vi "Create StateMachine.vi"(5 "statemachine in":refnum<class "statemachine.lvclass">, 8 "error in (no error)":errorcluster) -> (0 "error out":errorcluster, 3 "statemachine out":refnum<class "statemachine.lvclass">)   [LabVIEW 2020, in "eos.lvlib" / "statemachine.lvclass"]
uses:
  statemachine.lvclass
  interfaces/state/state.lvclass
  interfaces/initialization/initializable.lvclass
  C:/Projects/LVOS/EngineeringOS/source/interfaces/state/state.lvclass
  interfaces/data/data.lvclass
  statemachine.lvclass/statemachine.ctl
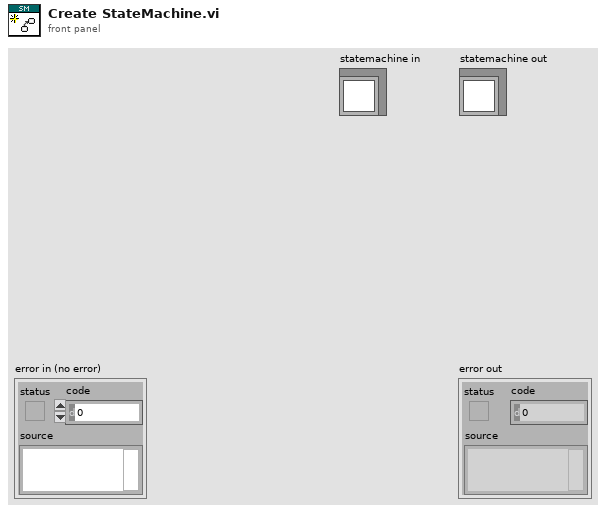
[diagram p1: front panel]
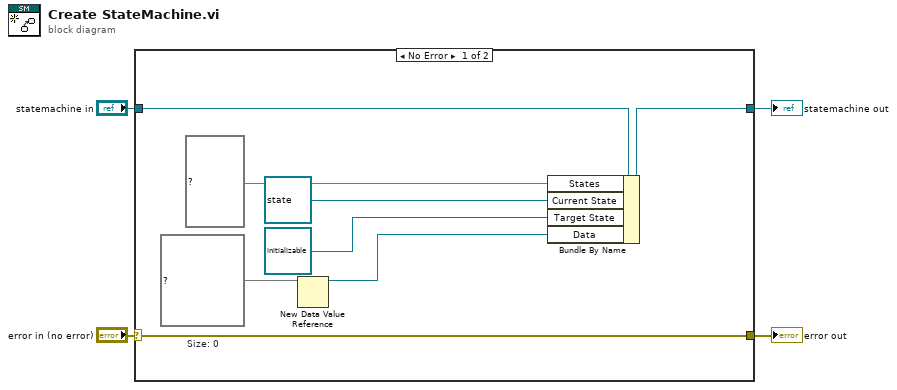
[diagram p0: block diagram]
diagram:
  n1 = case shown="No Error" "error in (no error)" {
    selector: "error in (no error)" -> [w12 w14]
    tunnel: [w12 w14] -> w3
    tunnel: [w9 w13] -> w1
    tunnel: "statemachine in" -> [w11 w13]
    frame No Error {
      w6 = map{string, refnum<class "data.lvclass">} {}  # Size: 0
      n2 = New Data Value Reference(data value=w6) -> (data value reference=w5:refnum<data-value>)  [unwired: 1 in, 1 out]
      n3 = Bundle By Name(cluster=w11, "States"=set{refnum<class "state.lvclass">} {} ("set"), "Current State"=refnum<class "state.lvclass"> refnum ("eos.lvlib:state.lvclass"), "Target State"=refnum<class "initializable.lvclass"> refnum ("eos.lvlib:initializable.lvclass"), "Data"=w5) -> (w9:refnum<class "statemachine.lvclass">)
    }
    frame Error {
    }
  }
  "error out" <- w3
  "statemachine out" <- w1
